vi "final cal y.vi"(0 "y0 base 1":dbl, 1 "y0 base 2":dbl, 2 "y0  base 3":dbl, 3 "d 1":dbl, 4 "d 2":dbl, 5 "d 3":dbl) -> (16 "y":dbl)   [LabVIEW 2026]
uses:
  <vilib>/express/express arith-compare/Formula/XNode/ExpressFormulaBlockNode.xnode
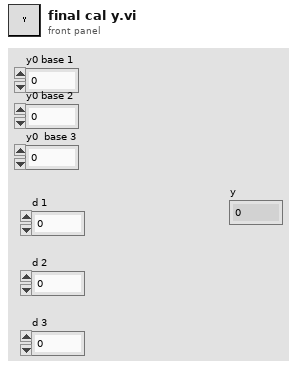
[diagram p1: front panel]
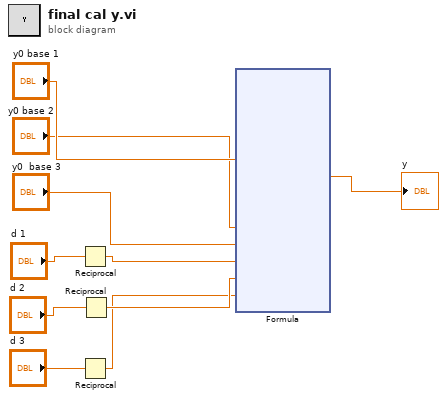
[diagram p0: block diagram]
diagram:
  n1 = Reciprocal(x="d 1") -> (1/x=w7:dbl)
  n2 = Reciprocal(x="d 3") -> (1/x=w5:dbl)
  n3 = Reciprocal(x="d 2") -> (1/x=w6:dbl)
  n4 = xnode "Formula"("y1"="y0 base 1", "y2"="y0 base 2", "y3"="y0  base 3", "w1"=w7, "w2"=w6, "w3"=w5) -> ("Result"=→"y":dbl)  [unwired: 1 in, 1 out]
